vi "manageJobData.vi"(5 "Action type":u16(ring)=1 items=["Delete", "Rename"], 7 "Storage location":u16(ring)=1 items=["Flash"=1, "USB"=2], 8 "error in (no error)":errorcluster, 9 "New file name":string="Test", 10 "Current file name":string="Test", 11 "SM1000-control in":T1) -> (0 "error out":errorcluster, 3 "SM1000-control out":T1)   [LabVIEW 2013, in "MaterialCharacterization.lvlib" / "MC-SM1000.lvclass"]
doc: "Manage jobs that have been stored on the EC1000.\n\nJobs already stored on the EC1000 can be renamed or deleted."
uses:
  MC-SM1000.lvclass
  Object-reference.ctl
  MC-SM1000.lvclass/MC-SM1000.ctl
  Custom-errors.ctl
  C:/Users/vangeste/Desktop/2015-06-02 - SLM - MAIF/HC-HardwareCharacterization/Sources/SM1000/LECSession.dll
  HC-HardwareCharacterization/Sources/SM1000/LECSession.dll
  DOTNET-error-int.vi
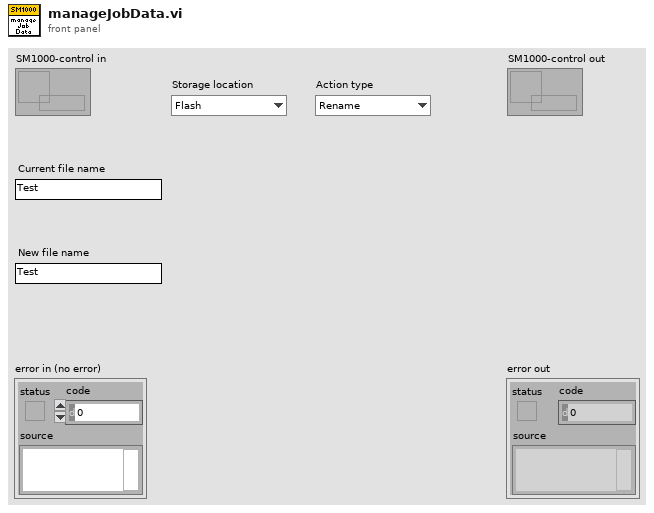
[diagram p1: front panel]
types:
  T1 = typedef "MaterialCharacterization.lvlib/MC-SM1000.lvclass/Object-reference.ctl" = refnum<data-value>
  T2 = typedef "MaterialCharacterization.lvlib/MC-SM1000.lvclass/Custom-errors.ctl" = enum16{"No error", "Not implemented", "Command not recognized", "Invalid input", "No connection", "Timeout", "Resource not loaded"}
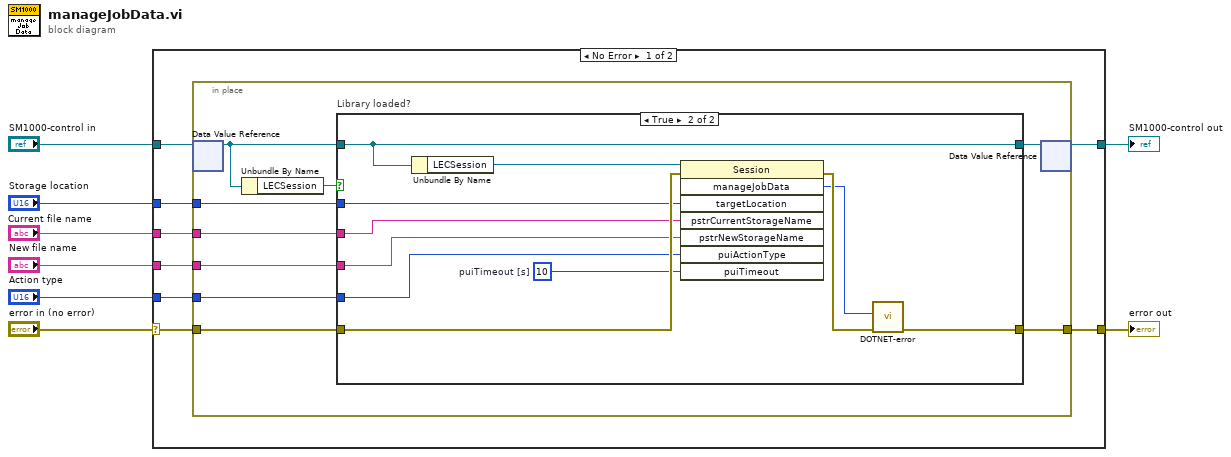
[diagram p0: block diagram]
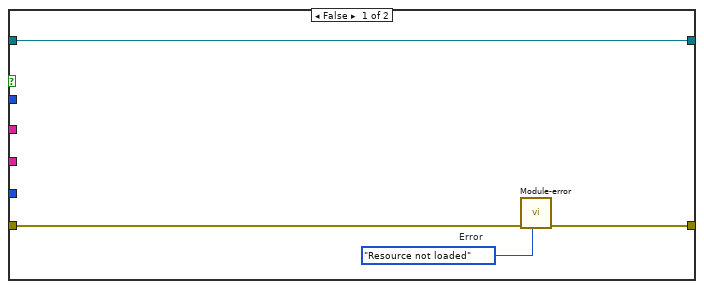
[diagram p2: hidden frame]
diagram:
  n1 = case shown="No Error" "error in (no error)" {
    selector: "error in (no error)" -> [w14 w42]
    tunnel: [w13 w42] -> w7
    tunnel: [w15 w41] -> w5
    tunnel: "SM1000-control in" -> [w16 w41]
    tunnel: "New file name" -> [w12 _]
    tunnel: "Action type" -> [w11 _]
    tunnel: "Storage location" -> [w10 _]
    tunnel: "Current file name" -> [w9 _]
    frame No Error {
      n2 = in-place {
        in-place-border: w14 -> [w25]
        in-place-border: [w22] -> w13
        in-place-border: w12 -> [w20]
        in-place-border: w11 -> [w19]
        in-place-border: w10 -> [w18]
        in-place-border: w9 -> [w17]
        n3 = in-place-dvr #1(w16) -> (w23:refnum<class "MC-SM1000.lvclass">)  [unwired: 1 out]
        n4 = Unbundle By Name(w23) -> ("LECSession"=w24:bool)
        n5 = case "Library loaded?" shown="True" w24 {
          tunnel: w25 -> [w29 w39]
          tunnel: w23 -> [w27 w38]
          tunnel: [w28 w32] -> w22
          tunnel: [w27 w38] -> w21
          tunnel: w20 -> [_ w34]
          tunnel: w19 -> [_ w35]
          tunnel: w18 -> [_ w37]
          tunnel: w17 -> [_ w33]
          frame False {
            w26 = Custom-errors."Resource not loaded"  # Error
            n6 = call "Module-error.vi"("Error"=w26, "error in (no error)"=w29) -> ("error out"=w28:errorcluster)  [unwired: 9 in]
          }
          frame True {
            w36 = u32 10  # puiTimeout [s]
            n7 = Unbundle By Name(w38) -> ("LECSession"=w40:refnum<k24>)
            n8 = invoke class="Session" method="manageJobData"(reference=w40, error in=w39, "targetLocation"=w37, "pstrCurrentStorageName"=w33, "pstrNewStorageName"=w34, "puiActionType"=w35, "puiTimeout"=w36) -> (error out=w31:errorcluster, "manageJobData"=w30:u32)  [unwired: 1 in, 6 out]
            n9 = call-poly "DOTNET-error.vi"("error in (no error)"=w31, "Retun code"=w30) -> ("error out"=w32:errorcluster)  [unwired: 9 in]
          }
        }
        n10 = in-place-dvr #1(w21) -> (w15:T1)  [unwired: 1 out]
      }
    }
    frame Error {
    }
  }
  "error out" <- w7
  "SM1000-control out" <- w5
